vi "3_1_PTLF_Classification_Eval(CPU,GPU).vi"() -> ()   [LabVIEW 2020]
doc: "This example demonstrates the usage of \"Deep Neural Network Accelerator for FPGA\" for Face detection and running for inference on RT targets using FPGA."
uses:
  <vilib>/Ngene/Deep Learning Toolkit/Toolkit/NN_Network/Controls/NN_Device.ctl
  <vilib>/Ngene/Deep Learning Toolkit/Toolkit/NN_Network/Controls/NN_Save_Before_Destroy_Options.ctl
  4973630c-52a8-4b5a-885b-d0de098afee9.vi
  <vilib>/Ngene/Deep Learning Toolkit/Toolkit/NN_Data/subVIs/Get_Data_Vals/2D/NN_Data_Get_ValByRef(2D_SGL).vi
  <vilib>/Ngene/Deep Learning Toolkit/Toolkit/NN_Data/subVIs/Dataset/NN_Variant_to_DVR/2D/NN_Data_Variant_to_DVR(2D_SGL).vi
  <vilib>/Ngene/Deep Learning Toolkit/Toolkit/NN_Data/subVIs/Get_Data_Vals/2D/NN_Data_Get_ValByRef(2D_SGL_idx).vi
  <vilib>/Ngene/Deep Learning Toolkit/Toolkit/NN_Network/API/NN_Set_Input/1D/NN_Set_Input(1D_SGL_idx).vi
  <vilib>/Ngene/Deep Learning Toolkit/Toolkit/NN_Train/Eval_Loss/NN_Eval_Test_Error_Loss/NN_Eval(In1D_Out1D).vi
  <vilib>/Ngene/Deep Learning Toolkit/Toolkit/NN_Train/Eval_Loss/NN_Calc_Cofusion_Matrix/NN_Calc_Confusion_Matrix(In1D_Out1D).vi
  <vilib>/Ngene/Deep Learning Toolkit/Toolkit/Deep_Learning_Toolkit_by_Ngene.lvlib
  <vilib>/ptbypt/NI_PtbyPt.lvlib
panel:
  in  "NN_Device":T1
  in  "Weight File Path":path=path "D:/Ngene/GitHub/deepltk_fpga_examples/3_PTLF_Classification(PXI,sbRIO)/Models/0_PTLF_Classification_Original/PTLF_Classifier_weights_24_11_21__13_37_15.bin"
  in  "Configuration File Path":path=path "D:/Ngene/GitHub/deepltk_fpga_examples/3_PTLF_Classification(PXI,sbRIO)/Models/0_PTLF_Classification_Original/PTLF_Classifier_net_cfg_24_11_21__13_37_15.cfg"
  out "Dataset Size":i32=1200
  out "Loop time(s)":dbl=0.0010359500000049592 format="%#_4p"
  out "Inference time(s)":dbl=0.001025560000061887 format="%#_4p"
  in  "Stop":bool
  out "Iterations":i32=1199
  in  "Dataset":path=path "D:/Ngene/GitHub/deepltk_fpga_examples/3_PTLF_Classification(PXI,sbRIO)/Dataset/Test"
  out "GT":string="Swell"
  out "Pred":string="Sag"
  in  "index":i32=5
  out "Incorectly Classified Sample":sgl[](graph)=[0.419, 0.429, 0.438, 0.446, 0.454, 0.462, 0.469, 0.475, 0.481, 0.487, 0.491, 0.495, 0.499, 0.502, 0.504, 0.506, 0.507, 0.508, 0.508, 0.508, 0.506, 0.505, 0.502, 0.499, 0.496, 0.492, 0.487, 0.482, 0.476, 0.47, 0.463, 0.456, 0.448, 0.439, 0.43, 0.421, 0.411, 0.4, 0.389, 0.378, 0.366, 0.354, 0.341, 0.328, 0.315, 0.301, 0.287, 0.272, 0.257, 0.242, 0.227, 0.211, 0.195, 0.179, 0.163, 0.146, 0.13, 0.113, 0.096, 0.079, 0.061, 0.044, 0.027, 0.01, -0.008, -0.025, -0.043, -0.06, -0.077, -0.094, -0.111, -0.128, -0.145, -0.161, -0.178, -0.194, -0.21, -0.225, -0.241, -0.256, -0.271, -0.285, -0.3, -0.313, -0.327, -0.34, -0.353, -0.365, -0.377, -0.388, -0.399, -0.41, -0.42, -0.429, -0.438, -0.447, -0.455, -0.462, -0.469, -0.652, -0.66, -0.667, -0.673, -0.679, -0.684, -0.688, -0.691, -0.694, -0.695, -0.696, -0.696, -0.695, -0.694, -0.691, -0.688, -0.684, -0.679, -0.674, -0.667, -0.66, -0.652, -0.643, -0.634, -0.624, -0.613, -0.601, -0.589, -0.576, -0.562, -0.548, -0.533, -0.517, -0.501, -0.484, -0.466, -0.449, -0.43, -0.411, -0.392, -0.372, -0.351, -0.331, -0.31, -0.288, -0.266, -0.244, -0.222, -0.199, -0.176, -0.153, -0.13, -0.106, -0.083, -0.059, -0.035, -0.012, 0.012, 0.036, 0.06, 0.083, 0.107, 0.13, 0.154, 0.177, 0.2, 0.222, 0.245, 0.267, 0.289, 0.31, 0.331, 0.352, 0.372, 0.392, 0.412, 0.43, 0.449, 0.467, 0.484, 0.501, 0.517, 0.533, 0.548, 0.562, 0.576, 0.589, 0.601, 0.613, 0.624, 0.634, 0.643, 0.652, 0.66, 0.667, 0.674, 0.679, 0.684, 0.688, 0.691, 0.694, 0.695, 0.696, 0.696, 0.695, 0.694, 0.691, 0.688, 0.684, 0.679, 0.673, 0.667, 0.659, 0.651, 0.643, 0.633, 0.623, 0.612, 0.6, 0.588, 0.575, 0.561, 0.547, 0.532, 0.516, 0.5, 0.483, 0.465, 0.447, 0.429, 0.41, 0.391, 0.371, 0.35, 0.329, 0.308, 0.287, 0.265, 0.243, 0.22, 0.198, 0.175, 0.152, 0.128, 0.105, 0.081, 0.058, 0.034, 0.01, -0.014, -0.037, -0.061, -0.085, -0.108, -0.132, -0.155, -0.178, -0.201, -0.224, -0.246, -0.268, -0.29, -0.311, -0.332, -0.353, -0.373, -0.393, -0.413, -0.432, -0.45, -0.468, -0.485, -0.502, -0.518, -0.534, -0.549, -0.563, -0.577, -0.59, -0.602, -0.614, -0.624, -0.635, -0.644, -0.653, -0.661, -0.668, -0.674, -0.68, -0.684, -0.688, -0.691, -0.694, -0.695, -0.696, -0.696, -0.695, -0.693, -0.691, -0.688, -0.683, -0.679, -0.673, -0.666, -0.659, -0.651, -0.642, -0.633, -0.622, -0.611, -0.6, -0.587, -0.574, -0.56, -0.546, -0.531, -0.515, -0.499, -0.482, -0.464, -0.446, -0.428, -0.409, -0.389, -0.369, -0.349, -0.328, -0.307, -0.286, -0.264, -0.242, -0.219, -0.196, -0.173, -0.15, -0.127, -0.104, -0.08, -0.056, -0.033, -0.009, 0.015, 0.039, 0.063, 0.086, 0.11, 0.133, 0.156, 0.131, 0.148, 0.164, 0.181, 0.197, 0.213, 0.228, 0.244, 0.259, 0.274, 0.288, 0.302, 0.316, 0.329, 0.342, 0.355, 0.367, 0.379, 0.39, 0.401, 0.412, 0.422, 0.431, 0.44, 0.448, 0.456, 0.464, 0.471, 0.477, 0.483, 0.488, 0.492, 0.496, 0.5, 0.503, 0.505, 0.507, 0.508, 0.508, 0.508, 0.507, 0.506, 0.504, 0.502, 0.499, 0.495, 0.491, 0.486, 0.481, 0.475, 0.468, 0.461, 0.454, 0.446, 0.437, 0.428, 0.418, 0.408, 0.398, 0.387, 0.375, 0.363, 0.351, 0.338, 0.325, 0.311, 0.298, 0.283, 0.269, 0.254, 0.239, 0.223, 0.207, 0.192, 0.175, 0.159, 0.142, 0.126, 0.109, 0.092, 0.075, 0.057, 0.04, 0.023, 0.005, -0.012, -0.029, -0.047, -0.064, -0.081, -0.098, -0.115, -0.132, -0.149, -0.165, -0.182, -0.198, -0.214, -0.229, -0.245, -0.26, -0.274, -0.289, -0.303, -0.317, -0.33, -0.343, -0.356, -0.368, -0.38, -0.391, -0.402, -0.412, -0.422, -0.432, -0.44, -0.449, -0.457, -0.464, -0.471, -0.477, -0.483, -0.488, -0.493, -0.497, -0.5, -0.503, -0.505, -0.507, -0.508, -0.508, -0.508, -0.507, -0.506, -0.504, -0.502, -0.499, -0.495, -0.491, -0.486, -0.48, -0.474, -0.468, -0.461, -0.453, -0.445, -0.437, -0.427, -0.418, -0.408, -0.397, -0.386, -0.375, -0.363, -0.35, -0.337, -0.324, -0.311, -0.297, -0.282, -0.268, -0.253, -0.238, -0.222, -0.207, -0.191, -0.174, -0.158, -0.141, -0.125, -0.108, -0.091, -0.074, -0.056, -0.039, -0.022, -0.004, 0.013, 0.03, 0.048, 0.065, 0.082, 0.099, 0.116, 0.133, 0.15, 0.166, 0.183, 0.199, 0.214, 0.23, 0.245, 0.261, 0.275, 0.29, 0.304, 0.318, 0.331, 0.344, 0.356, 0.369, 0.38, 0.392, 0.402, 0.413, 0.423, 0.432, 0.441, 0.449, 0.457, 0.465, 0.471, 0.478, 0.483, 0.488, 0.493, 0.497, 0.5, 0.503, 0.505, 0.507, 0.508, 0.508, 0.508, 0.507, 0.506, 0.504, 0.501, 0.498, 0.495, 0.49, 0.485, 0.48, 0.474, 0.468, 0.46, 0.453, 0.445, 0.436, 0.427, 0.417, 0.407, 0.396, 0.385, 0.374, 0.362, 0.349, 0.337, 0.323, 0.31, 0.296, 0.282, 0.267, 0.252, 0.237, 0.221, 0.206, 0.19, 0.173, 0.157, 0.14, 0.124, 0.107, 0.09, 0.072, 0.055, 0.038, 0.021, 0.003, -0.014, -0.031, -0.049, -0.066, -0.083, -0.1, -0.117, -0.134, -0.151, -0.167, -0.183, -0.2, -0.215, -0.231, -0.246, -0.261, -0.276, -0.291, -0.305, -0.318, -0.332, -0.345, -0.357, -0.369, -0.381, -0.392, -0.403, -0.413, -0.423, -0.433, -0.442, -0.45, -0.458, -0.465, -0.472, -0.478, -0.484, -0.489, -0.493, -0.497, -0.5, -0.503, -0.505, -0.507, -0.508, -0.508, -0.508, -0.507, -0.506, -0.504, -0.501, -0.498, -0.494, -0.49, -0.485, -0.48, -0.474, -0.467, -0.46, -0.452, -0.444, -0.436, -0.426, -0.417, -0.406, -0.396, -0.385, -0.373, -0.361, -0.349, -0.336, -0.323, -0.309, -0.295, -0.281, -0.266, -0.251, -0.236, -0.22, -0.205, -0.189, -0.172, -0.156, -0.139, -0.123, -0.106, -0.089, -0.071, -0.054, -0.037, -0.02, -0.002, 0.015, 0.032, 0.05, 0.067, 0.084, 0.101, 0.118, 0.135, 0.152, 0.168, 0.184, 0.201, 0.216, 0.232, 0.247, 0.262, 0.277, 0.291, 0.305, 0.319, 0.332, 0.345, 0.358, 0.37, 0.382, 0.393, 0.404, 0.414, 0.424, 0.433, 0.442, 0.45, 0.458, 0.465, 0.472, 0.478, 0.484, 0.489, 0.493, 0.497, 0.5, 0.503, 0.505, 0.507, 0.508, 0.508, 0.508, 0.507, 0.506, 0.504, 0.501, 0.498, 0.494, 0.49, 0.485, 0.479, 0.473, 0.467, 0.46, 0.452, 0.444, 0.435, 0.426, 0.416, 0.406, 0.395, 0.384, 0.372, 0.36, 0.348, 0.335, 0.322, 0.308, 0.294, 0.28, 0.265, 0.25, 0.235, 0.219, 0.204, 0.188, 0.171, 0.155, 0.138, 0.122, 0.105, 0.088, 0.07, 0.053, 0.036, 0.019, 0.001, -0.016, -0.034, -0.051, -0.068, -0.085, -0.102, -0.119, -0.136, -0.153, -0.169, -0.185, -0.201, -0.217, -0.233, -0.248, -0.263, -0.278, -0.292, -0.306, -0.32, -0.333, -0.346, -0.359, -0.371, -0.382, -0.394, -0.404, -0.415, -0.424, -0.434, -0.443, -0.451, -0.459, -0.466, -0.472, -0.479, -0.484, -0.489, -0.494, -0.497, -0.501, -0.503, -0.505, -0.507, -0.508, -0.508, -0.508, -0.507, -0.506, -0.504, -0.501, -0.498, -0.494, -0.49, -0.485, -0.479, -0.473, -0.466, -0.459, -0.451, -0.443, -0.434, -0.425, -0.415, -0.405, -0.394, -0.383, -0.372, -0.36, -0.347, -0.334, -0.321, -0.307, -0.293, -0.279, -0.264, -0.249, -0.234, -0.219, -0.203, -0.187, -0.17, -0.154, -0.137, -0.121, -0.104, -0.087, -0.069, -0.052, -0.035, -0.018, -0.0, 0.017, 0.035, 0.052, 0.069, 0.086, 0.103, 0.12, 0.137, 0.154, 0.17, 0.186, 0.202, 0.218, 0.234, 0.249, 0.264, 0.279, 0.293, 0.307, 0.321, 0.334, 0.347, 0.359, 0.371, 0.383, 0.394, 0.405, 0.415, 0.425, 0.434, 0.443, 0.451, 0.459, 0.466, 0.473, 0.479, 0.484, 0.489, 0.494, 0.498, 0.501, 0.504, 0.506, 0.507, 0.508, 0.508, 0.508, 0.507, 0.505, 0.503, 0.501, 0.497, 0.494, 0.489, 0.484, 0.479, 0.473, 0.466, 0.459, 0.451, 0.443, 0.434, 0.425, 0.415, 0.405, 0.394, 0.383, 0.371, 0.359, 0.346, 0.333, 0.32, 0.307, 0.292, 0.278, 0.263, 0.248, 0.233, 0.218, 0.202, 0.186, 0.169, 0.153, 0.136, 0.12, 0.103, 0.086, 0.068, 0.051, 0.034, 0.016, -0.001, -0.018, -0.036, -0.053, -0.07, -0.087, -0.104, -0.121, -0.138, -0.155, -0.171, -0.187, -0.203, -0.219, -0.235, -0.25, -0.265, -0.28, -0.294, -0.308, -0.322, -0.335, -0.348, -0.36, -0.372, -0.384, -0.395, -0.406, -0.416, -0.426, -0.435, -0.444, -0.452, -0.459, -0.467, -0.473, -0.479, -0.485, -0.49, -0.494, -0.498, -0.501, -0.504, -0.506, -0.507, -0.508, -0.508, -0.508, -0.507, -0.505, -0.503, -0.501, -0.497, -0.493, -0.489, -0.484, -0.478, -0.472, -0.465, -0.458, -0.45, -0.442, -0.433, -0.424, -0.414, -0.404, -0.393, -0.382, -0.37, -0.358, -0.346, -0.333, -0.319, -0.306, -0.292, -0.277, -0.263, -0.248, -0.232, -0.217, -0.201, -0.185, -0.168, -0.152, -0.135, -0.119, -0.102, -0.084, -0.067, -0.05, -0.033, -0.015, 0.002, 0.019, 0.037, 0.054, 0.071, 0.088, 0.105, 0.122, 0.139, 0.156, 0.172, 0.188, 0.204, 0.22, 0.236, 0.251, 0.266, 0.28, 0.295, 0.309, 0.322, 0.336, 0.348, 0.361, 0.373, 0.384, 0.396, 0.406, 0.416, 0.426, 0.435, 0.444, 0.452, 0.46, 0.467, 0.474, 0.48, 0.485, 0.49, 0.494, 0.498, 0.501, 0.504, 0.506, 0.507, 0.508, 0.508, 0.508, 0.507, 0.505, 0.503, 0.5, 0.497, 0.493, 0.489, 0.484, 0.478, 0.472, 0.465, 0.458, 0.45, 0.442, 0.433, 0.423, 0.414, 0.403, 0.393, 0.381, 0.37, 0.357, 0.345, 0.332, 0.319, 0.305, 0.291, 0.276, 0.262, 0.247, 0.231, 0.216, 0.2, 0.184, 0.167, 0.151, 0.134, 0.117, 0.101, 0.083, 0.066, 0.049, 0.032, 0.014, -0.003, -0.02, -0.038, -0.055, -0.072, -0.089, -0.106, -0.123, -0.14, -0.157, -0.173, -0.189, -0.205, -0.221, -0.237, -0.252, -0.267, -0.281, -0.296, -0.31, -0.323, -0.336, -0.349, -0.362, -0.374, -0.385, -0.396, -0.407, -0.417, -0.427, -0.436, -0.445, -0.453, -0.46, -0.467, -0.474, -0.48, -0.485, -0.49, -0.495, -0.498, -0.501, -0.504, -0.506, -0.507, -0.508, -0.508, -0.508, -0.507, -0.505, -0.503, -0.5, -0.497, -0.493, -0.488, -0.483, -0.478, -0.471, -0.465, -0.457, -0.45, -0.441, -0.432, -0.423, -0.413, -0.403, -0.392, -0.381, -0.369, -0.357, -0.344, -0.331, -0.318, -0.304, -0.29, -0.276, -0.261, -0.246, -0.23, -0.215, -0.199, -0.183, -0.166, -0.15, -0.133, -0.116, -0.1, -0.082, -0.065, -0.048, -0.031, -0.013, 0.004, 0.021, 0.039, 0.056, 0.073, 0.09, 0.107, 0.124, 0.141, 0.158, 0.174, 0.19, 0.206, 0.222, 0.238, 0.253, 0.268, 0.282, 0.297, 0.31, 0.324, 0.337, 0.35, 0.362, 0.374, 0.386, 0.397, 0.408, 0.418, 0.427, 0.436, 0.445, 0.453, 0.461, 0.468, 0.474, 0.48, 0.486, 0.491, 0.495, 0.498, 0.502, 0.504, 0.506, 0.507, 0.508, 0.508, 0.508, 0.507, 0.505, 0.503, 0.5, 0.497, 0.493, 0.488, 0.483, 0.477, 0.471, 0.464, 0.457, 0.449, 0.441, 0.432, 0.422, 0.412, 0.402, 0.391, 0.38, 0.368, 0.356, 0.343, 0.33, 0.317, 0.303, 0.289, 0.275, 0.26, 0.245, 0.229, 0.214, 0.198, 0.182, 0.166, 0.149, 0.132, 0.115, 0.098, 0.081, 0.064, 0.047, 0.03, 0.012, -0.005, -0.022, -0.04, -0.057, -0.074, -0.091, -0.108, -0.125, -0.142, -0.159, -0.175, -0.191, -0.207, -0.223, -0.238, -0.254, -0.269, -0.283, -0.297, -0.311, -0.325, -0.338, -0.351, -0.363, -0.375, -0.387, -0.398, -0.408, -0.418, -0.428, -0.437, -0.446, -0.454, -0.461, -0.468, -0.475, -0.481, -0.486, -0.491, -0.495, -0.499, -0.502, -0.504, -0.506, -0.507, -0.508, -0.508, -0.508, -0.507, -0.505, -0.503, -0.5, -0.496, -0.492, -0.488, -0.483, -0.477, -0.471, -0.464, -0.456, -0.449, -0.44, -0.431, -0.422, -0.412, -0.401, -0.391, -0.379, -0.367, -0.355, -0.343, -0.33, -0.316, -0.302, -0.288, -0.274, -0.259, -0.244, -0.228, -0.213, -0.197, -0.181, -0.165, -0.148, -0.131, -0.114, -0.097, -0.08, -0.063, -0.046, -0.029, -0.011, 0.006, 0.023, 0.041, 0.058, 0.075, 0.092, 0.109, 0.126, 0.143, 0.16, 0.176, 0.192, 0.208, 0.224, 0.239, 0.255, 0.269, 0.284, 0.298, 0.312, 0.326, 0.339, 0.351, 0.364, 0.376, 0.387, 0.398, 0.409, 0.419, 0.428, 0.438, 0.446, 0.454, 0.462, 0.469, 0.475, 0.481, 0.486, 0.491, 0.495, 0.499, 0.502, 0.504, 0.506, 0.507, 0.508, 0.508, 0.508, 0.507, 0.505, 0.503, 0.5, 0.496, 0.492, 0.487, 0.482, 0.477, 0.47, 0.463, 0.456, 0.448, 0.44, 0.431, 0.421, 0.411, 0.401, 0.39, 0.378, 0.367, 0.354, 0.342, 0.329, 0.315, 0.302, 0.287, 0.273, 0.258, 0.243, 0.228, 0.212, 0.196, 0.18, 0.164, 0.147, 0.13, 0.113, 0.096, 0.079, 0.062, 0.045, 0.028, 0.01, -0.007, -0.025, -0.042, -0.059, -0.076, -0.093, -0.11, -0.127, -0.144, -0.161, -0.177, -0.193, -0.209, -0.225, -0.24, -0.255, -0.27, -0.285, -0.299, -0.313, -0.326, -0.34, -0.352, -0.365, -0.376, -0.388, -0.399, -0.409, -0.419, -0.429, -0.438, -0.447, -0.455, -0.462, -0.469, -0.475, -0.481, -0.487, -0.491, -0.495, -0.499, -0.502, -0.504, -0.506, -0.507, -0.508, -0.508, -0.508, -0.506, -0.505, -0.502, -0.499, -0.496, -0.492, -0.487, -0.482, -0.476, -0.47, -0.463, -0.456, -0.448, -0.439, -0.43, -0.421, -0.411, -0.4, -0.389, -0.378, -0.366, -0.354, -0.341, -0.328, -0.314, -0.301, -0.286, -0.272, -0.257, -0.242, -0.227, -0.211, -0.195, -0.179, -0.163, -0.146, -0.129, -0.112, -0.095, -0.078, -0.061, -0.044, -0.027, -0.009, 0.008, 0.026, 0.043, 0.06, 0.077, 0.094, 0.111, 0.128, 0.145, 0.162, 0.178, 0.194, 0.21, 0.226, 0.241, 0.256, 0.271, 0.286, 0.3, 0.314, 0.327, 0.34, 0.353, 0.365, 0.377, 0.389, 0.4, 0.41, 0.42, 0.43, 0.439, 0.447, 0.455, 0.463, 0.469, 0.476, 0.482, 0.487, 0.492, 0.496, 0.499, 0.502, 0.505, 0.506, 0.508, 0.508, 0.508, 0.508, 0.506, 0.505, 0.502, 0.499, 0.496, 0.492, 0.487, 0.482, 0.476, 0.469, 0.463, 0.455, 0.447, 0.439, 0.43, 0.42, 0.41, 0.399, 0.389, 0.377, 0.365, 0.353, 0.34, 0.327, 0.314, 0.3, 0.286, 0.271, 0.256, 0.241, 0.226, 0.21, 0.194, 0.178, 0.162, 0.145, 0.128, 0.111, 0.094, 0.077, 0.06, 0.043, 0.025, 0.008, -0.009, -0.027, -0.044, -0.061, -0.078, -0.095, -0.112, -0.129, -0.146, -0.163, -0.179, -0.195, -0.211, -0.227, -0.242, -0.257, -0.272, -0.287, -0.301, -0.315, -0.328, -0.341, -0.354, -0.366, -0.378, -0.389, -0.4, -0.411, -0.421, -0.43, -0.439, -0.448, -0.456, -0.463, -0.47, -0.476, -0.482, -0.487, -0.492, -0.496, -0.499, -0.502, -0.505, -0.506, -0.508, -0.508, -0.508, -0.507, -0.506, -0.504, -0.502, -0.499, -0.495, -0.491, -0.487, -0.481, -0.475, -0.469, -0.462, -0.455, -0.447, -0.438, -0.429, -0.419, -0.409, -0.399, -0.388, -0.376, -0.364, -0.352, -0.339, -0.326, -0.313, -0.299, -0.285, -0.27, -0.255, -0.24, -0.225, -0.209, -0.193, -0.177, -0.161, -0.144, -0.127, -0.11, -0.093, -0.076, -0.059, -0.042, -0.024, -0.007, 0.01, 0.028, 0.045, 0.062, 0.079, 0.097, 0.114, 0.13, 0.147, 0.164, 0.18, 0.196, 0.212, 0.228, 0.243, 0.258, 0.273, 0.287, 0.302, 0.315, 0.329, 0.342, 0.354, 0.367, 0.379, 0.39, 0.401, 0.411, 0.421, 0.431, 0.44, 0.448, 0.456, 0.463, 0.47, 0.477, 0.482, 0.488, 0.492, 0.496, 0.5, 0.503, 0.505, 0.507, 0.508, 0.508, 0.508, 0.507, 0.506, 0.504, 0.502, 0.499, 0.495, 0.491, 0.486, 0.481, 0.475, 0.469, 0.462, 0.454, 0.446, 0.437, 0.428, 0.419, 0.409, 0.398, 0.387, 0.376, 0.364, 0.351, 0.339, 0.326, 0.312, 0.298, 0.284, 0.269, 0.254, 0.239, 0.224, 0.208, 0.192, 0.176, 0.16, 0.143, 0.126, 0.109, 0.092, 0.075, 0.058, 0.041, 0.023, 0.006, -0.011, -0.029, -0.046, -0.063, -0.08, -0.098, -0.115, -0.131, -0.148, -0.165, -0.181, -0.197, -0.213, -0.229, -0.244, -0.259, -0.274, -0.288, -0.302, -0.316, -0.33, -0.343, -0.355, -0.367, -0.379, -0.391, -0.401, -0.412, -0.422, -0.431, -0.44, -0.449, -0.456, -0.464, -0.471, -0.477, -0.483, -0.488, -0.492, -0.496, -0.5, -0.503, -0.505, -0.507, -0.508, -0.508, -0.508, -0.507, -0.506, -0.504, -0.502, -0.499, -0.495, -0.491, -0.486, -0.481, -0.475, -0.468, -0.461, -0.454, -0.446, -0.437, -0.428, -0.418, -0.408, -0.398, -0.386, -0.375, -0.363, -0.351, -0.338, -0.325, -0.311, -0.297, -0.283, -0.268, -0.254, -0.238, -0.223, -0.207, -0.191, -0.175, -0.159, -0.142, -0.125, -0.108, -0.091, -0.074, -0.057, -0.04, -0.022, -0.005, 0.012, 0.03, 0.047, 0.064, 0.081]
  out "Confusion Matrix (Table)":string[][](table)=[["200", "0", "0", "0", "0", "0", "1.0000"], ["0", "199", "0", "1", "0", "0", "0.9950"], ["0", "0", "200", "0", "0", "0", "1.0000"], ["0", "0", "1", "197", "2", "0", "0.9850"], ["0", "0", "1", "23", "176", "0", "0.8800"], ["0", "0", "0", "0", "0", "200", "1.0000"], ["1.0000", "1.0000", "0.9901", "0.8914", "0.9888", "1.0000", ""]]
  out "Error":sgl=0.023333333
  out "Loss":sgl=0.061028734
  # "Overview: This VI is designed to evaluate (measure the accuracy of) the model when executed on CPU or GPU.\nRequirements: \n•DeepLTK - Deep Learning Toolkit for LabVIEW (https://www.ngene.co/deep-learning-toolkit-for-labview)\nInstructions:\n1.\tProvide the path to the dataset to be evaluated at Dataset control. \n2.\tProvide the \"Network Configuration File Path\" and \"Weight File Path\" generated by 1_PTLF_Classification_Training.vi or sample from project (locted in \"Models\\1_PTLF_Classification_Original\" folder.\n3.Use NN_Device to specify the device (CPU or GPU) for execution. GPU is applicable only for 64-bit LabVIEW.\n4. Run the VI with the default remaining settings.\n5. Observe mersured accuracy at Loss, Error and Confusion Matrix indicators, and analyze Incorectly Classified Sample by selecting samples with help of index control.\n6. Press the Stop button to stop the VI. \nMore Examples: https://github.com/ngenehub/deepltk_fpga_examples"
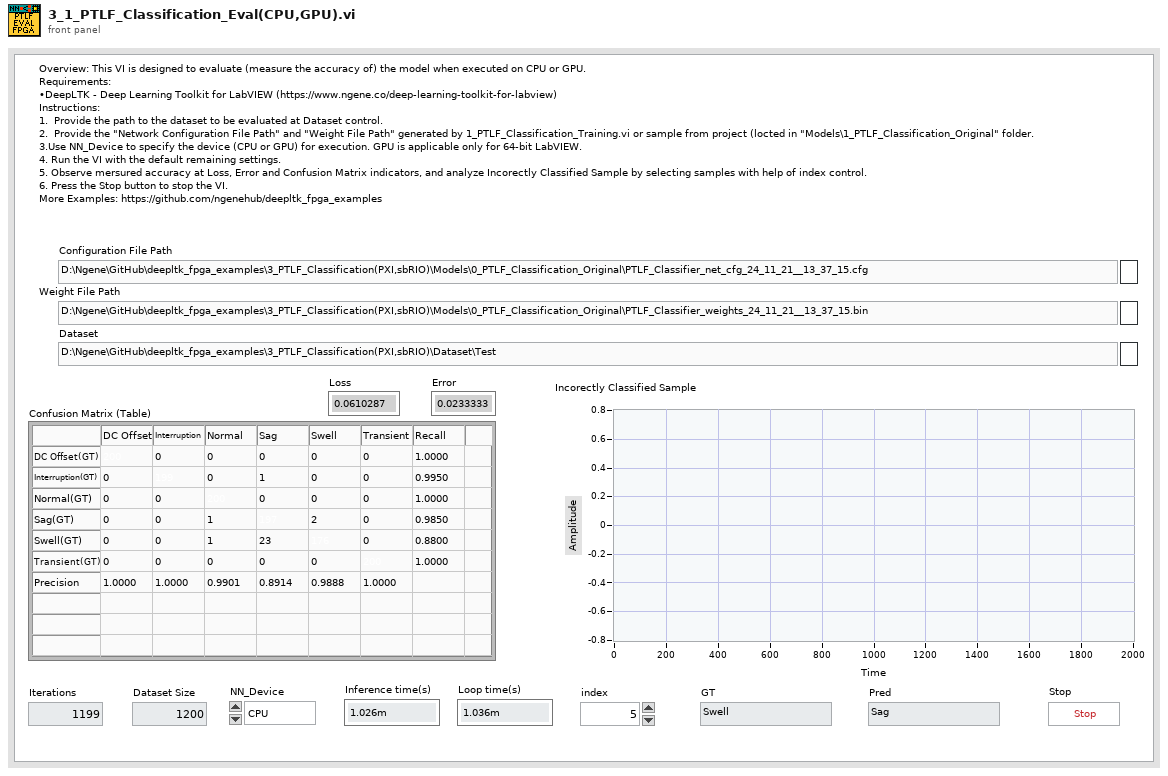
[diagram p1: front panel]
types:
  T1 = typedef "Deep_Learning_Toolkit_by_Ngene.lvlib/NN_Device.ctl" = enum16{"CPU", "GPU"}
  T2 = typedef "Deep_Learning_Toolkit_by_Ngene.lvlib/NN_Save_Before_Destroy_Options.ctl" = cluster{"CFG?":bool, "Weights?":bool, "Render?":bool}
  T3 = typedef "Deep_Learning_Toolkit_by_Ngene.lvlib/NN_DataSets_All(In1D_Out1D).ctl" = cluster{"Train":T4, "Validation":T4, "Test":T4}
  T4 = typedef "Deep_Learning_Toolkit_by_Ngene.lvlib/NN_DataSet(In1D_Out1D).ctl" = cluster{"Inputs Ref.":variant, "Outputs Ref.":T5, "Dims_In":i32, "Dataset_Size":i32, "Dims_Out":i32, "Labels":string[], "File Paths":path[]}
  T5 = typedef "Deep_Learning_Toolkit_by_Ngene.lvlib/NN_Data_ref(2D_SGL).ctl" = refnum<data-value>
  T6 = typedef "Deep_Learning_Toolkit_by_Ngene.lvlib/NN_Config_Params.ctl" = cluster{"Name":string, "mBatch":i32, "NN_Train_Params":T7, "LR_Decay_Policy":T10, "Labels":string[], "Loss":T12}
  T7 = typedef "Deep_Learning_Toolkit_by_Ngene.lvlib/NN_Train_Params.ctl" = cluster{"Optimizer":T8, "Beta_1":sgl, "Beta_2":sgl, "Weight Decay(L1)":sgl, "Weight Decay(L2)":sgl, "Data_Sampling":T9}
  T8 = typedef "Deep_Learning_Toolkit_by_Ngene.lvlib/NN_Train_Optimizer.ctl" = enum16{"SGD", "Adam", "Adagrad", "Adadelta", "RMSProp", "Nesterov"}
  T9 = typedef "Deep_Learning_Toolkit_by_Ngene.lvlib/NN_Train_Data_Sampling.ctl" = enum16{"Random", "Sequential"}
  T10 = typedef "Deep_Learning_Toolkit_by_Ngene.lvlib/NN_LR_Policy_Cfg.ctl" = cluster{"Policy_Type":T11, "LR0":dbl, "k":sgl, "WarmUp_Policy":enum16{"Step", "Ramp"}, "WarmUp_Iter":i32, "WarmUp_Ratio":sgl}
  T11 = typedef "Deep_Learning_Toolkit_by_Ngene.lvlib/NN_LR_Policy_Type.ctl" = enum16{"Manual", "Step", "Exp", "1/t"}
  T12 = typedef "Deep_Learning_Toolkit_by_Ngene.lvlib/NN_Loss_Config_Params.ctl" = cluster{"Loss_Type":T13, "Loss_Conf_Params":variant}
  T13 = typedef "Deep_Learning_Toolkit_by_Ngene.lvlib/NN_Loss_Type.ctl" = enum16{"None", "MSE", "CrossEntropy", "YOLO_v2", "YOLO_v4"}
  T14 = typedef "Deep_Learning_Toolkit_by_Ngene.lvlib/NN_Layer_Config_Params.ctl" = cluster{"Layer_Type":T15, "Layer_Conf_Params":variant, "Input Layers":string[]}
  T15 = typedef "Deep_Learning_Toolkit_by_Ngene.lvlib/NN_Layer_Type.ctl" = enum16{"Input1D", "Input3D", "Conv1D", "Conv2D", "Conv2D_Adv", "MaxPool", "AvgPool", "UpSample", "DropOut3D", "ShortCut", "Concat", "SoftMax3D", "FC", "DropOut", "Softmax", "Flatten", "YOLO_v2", "YOLO_v4", "Activation", "BatchNormalization", "Unsupported"}
  T16 = typedef "Deep_Learning_Toolkit_by_Ngene.lvlib/NN.ctl" = cluster{"Name":string, "No of Layers":i32, "mBatch":i32, "Layers":T17[], "Dimty":T18, "Dims_In":T19, "Dims_Out":T19, "Working_Dir":path, "Train?":bool, "Train_Params":T7, "LR_Update_Policy":T10, "Session Data":T20, "Ground_truth":T21, "NNg_hdls":T22, "NN_Device":T1, "GPU Id":i32, "Labels":string[], "Receptive Field":T23[], "Loss_Type":T13, "Loss_Cfg_Prms":variant, "NNG_WS":T24}
  T17 = typedef "Deep_Learning_Toolkit_by_Ngene.lvlib/NN_Layer_ref.ctl" = refnum<data-value>
  T18 = typedef "Deep_Learning_Toolkit_by_Ngene.lvlib/NN_In_Out_Dim-ty.ctl" = enum8{"In1D_Out1D", "In3D_Out1D", "In3D_Out3D", "In3D_OutBBox"}
  T19 = typedef "Deep_Learning_Toolkit_by_Ngene.lvlib/NN_Dims(C,H,W).ctl" = cluster{"C":i32, "H":i32, "W":i32}
  T20 = typedef "Deep_Learning_Toolkit_by_Ngene.lvlib/NN_Train_Session_Data.ctl" = cluster{"Epochs":sgl, "Tot_Iter":i32, "LR":sgl, "LR_iter":i32}
  T21 = typedef "Deep_Learning_Toolkit_by_Ngene.lvlib/NN_Ground_truth.ctl" = cluster{"Y":variant}
  T22 = typedef "Deep_Learning_Toolkit_by_Ngene.lvlib/nng_cuda_handles.ctl" = cluster{"cudnn":u64, "cublas":u64, "stream":u64, "curand":u64}
  T23 = typedef "Deep_Learning_Toolkit_by_Ngene.lvlib/NN_Dims(V,H).ctl" = cluster{"V":i32, "H":i32}
  T24 = typedef "Deep_Learning_Toolkit_by_Ngene.lvlib/NNG_WS.ctl" = cluster{"NNG_WS_Mem":T25, "Max_WS_Size":i64}
  T25 = typedef "Deep_Learning_Toolkit_by_Ngene.lvlib/NNg_WS_Mem_DVR.ctl" = refnum<data-value>
  T26 = typedef "Deep_Learning_Toolkit_by_Ngene.lvlib/NN_Layer.ctl" = cluster{"Name":string, "Layer_Data":variant, "Layer_Type":T15, "Dims_In":T19, "Layers_In":variant, "Dims_Out":T19, "Layers_Out":variant, "Metrics":T27, "GPU_Data":variant, "mBatch":i32, "NN_Device":T1, "NNg_hdls":T22, "Train?":bool, "Dimty":T28, "RecptField":T29}
  T27 = typedef "Deep_Learning_Toolkit_by_Ngene.lvlib/NN_Layer_Metrics.ctl" = cluster{"Data":dbl, "Params":dbl, "Ops":dbl}
  T28 = typedef "Deep_Learning_Toolkit_by_Ngene.lvlib/NN_Layer_Dimty.ctl" = enum16{"1D", "3D"}
  T29 = typedef "Deep_Learning_Toolkit_by_Ngene.lvlib/NN_Layer_RF_State.ctl" = cluster{"Dims":T23, "J":T23}
  T30 = typedef "Deep_Learning_Toolkit_by_Ngene.lvlib/NN_Eval_Params.ctl" = cluster{"Loss":sgl, "Error":sgl}
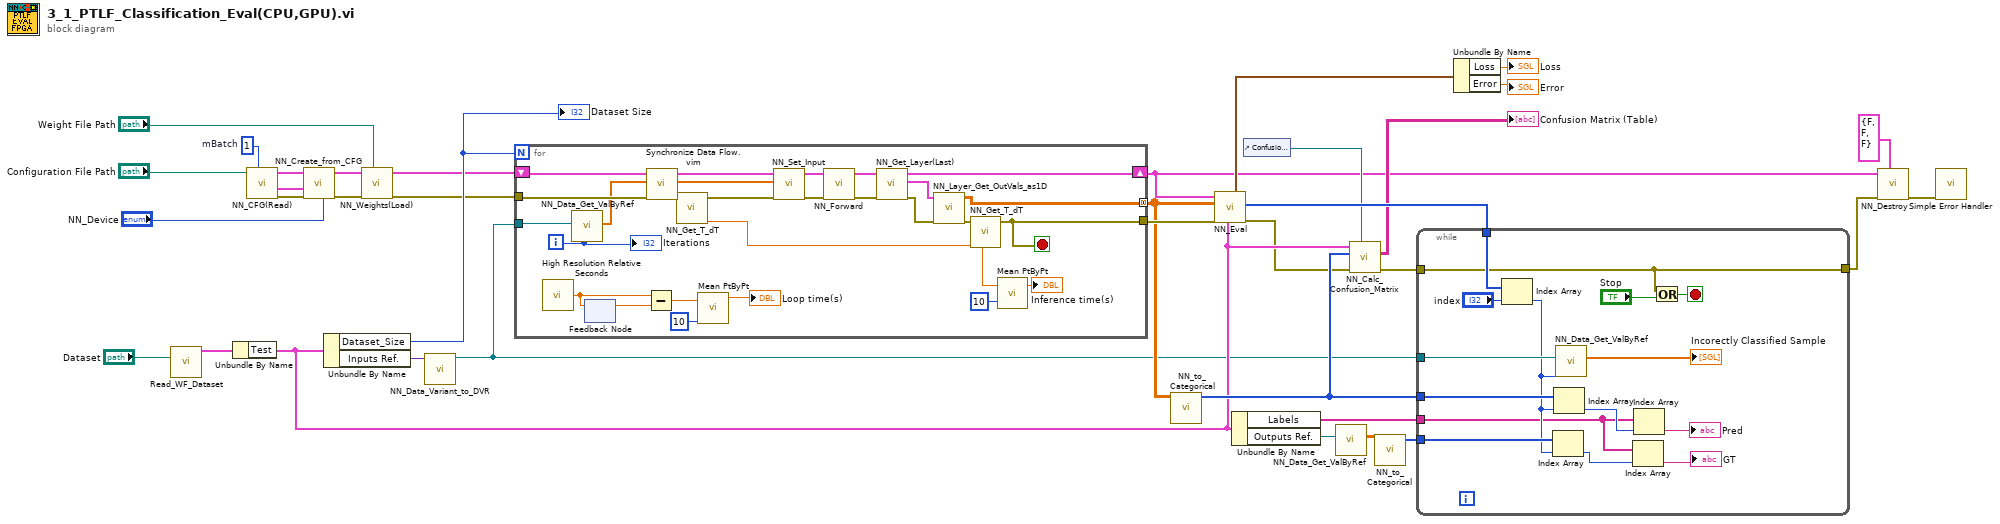
[diagram p0: block diagram]
diagram:
  w7 = 1  # mBatch
  n1 = call "Read_WF_Dataset.vi"("Test dataset path"="Dataset") -> ("NN_Dataset"=w24:T3)  [unwired: 10 in]
  n2 = Unbundle By Name(w24) -> ("Test"=w23:T4)
  n3 = call <vilib>:"NN_CFG(Read).vi"("mBatch"=w7, "CFG file path"="Configuration File Path") -> ("error out"=w10:errorcluster, "Net_Cfg"=w11:T6, "Layer_Cfg"=w9:T14[])  [unwired: 7 in]
  n4 = call <vilib>:"NN_Create_from_CFG.vi"("NN_Device"="NN_Device", "error in (no error)"=w10, "Net_Cfg"=w11, "Layer_Cfg"=w9) -> ("error out"=w12:errorcluster, "NN out"=w8:T16)  [unwired: 6 in]
  n5 = Unbundle By Name(w23) -> ("Dataset_Size"=w16:i32, "Inputs Ref."=w35:variant)
  "Dataset Size" <- w16
  n6 = call <vilib>:"NN_Weights(Load).vi"("Weight File Path"="Weight File Path", "error in (no error)"=w12, "NN in"=w8) -> ("error out"=w3:errorcluster, "NN out"=w4:T16)  [unwired: 7 in]
  n7 = call-poly <vilib>:"NN_Data_Variant_to_DVR.vi"("Inputs Ref."=w35) -> ("DVR(2D_SGL)"=w14:T5)  [unwired: 9 in, 1 out]
  n8 = for {
    N: w16 -> [_]
    shift-right: [w38] -> w15
    shift-left: w4 -> [w54]
    tunnel: w14 -> [w64]
    tunnel: [w59] -> w29 mode=concatenating
    tunnel: [w47] -> w34
    tunnel: w3 -> [w53]
    i -> [w58]
    stop <- w47 stop-if-true
    n9 = call <vilib>:"High Resolution Relative Seconds.vi"() -> ("relative seconds"=w55:dbl)
    n10 = call-poly <vilib>:"NN_Data_Get_ValByRef.vi"("index (row)"=w58, "DVR(2D_SGL)"=w64) -> ("Value(1D_SGL)"=w51:sgl[])  [unwired: 6 in, 1 out]
    n11 = feedback #1() -> (w56:dbl)  [unwired: 1 in]
    n12 = feedback-in #1(w55) -> ()
    n13 = Subtract(x=w55, y=w56) -> (x-y=w57:dbl)
    n14 = call "Synchronize Data Flow.vim"("input 4"=w53, "input 2"=w51, "input 1"=w54) -> ("output 4"=w52:errorcluster, "output 2"=w49:sgl[], "output 1"=w50:T16)  [unwired: 1 in, 1 out]
    n15 = call <vilib>:"NN_Get_T_dT.vi"("error in (no error)"=w52) -> ("T_out"=w46:dbl, "error out"=w48:errorcluster)  [unwired: 6 in, 1 out]
    n16 = call <vilib>:"Mean PtByPt.vi"("x"=w57, "sample length"=10) -> ("mean"=→"Loop time(s)":dbl)  [unwired: 2 in, 1 out]
    n17 = call-poly <vilib>:"NN_Set_Input.vi"("error in (no error)"=w48, "Data_In(1D_SGL)"=w49, "NN In"=w50) -> ("error out"=w62:errorcluster, "NN Out"=w63:T16)  [unwired: 7 in]
    n18 = call <vilib>:"NN_Forward.vi"("error in (no error)"=w62, "NN in"=w63) -> ("error out"=w61:errorcluster, "NN out"=w39:T16)  [unwired: 6 in, 2 out]
    n19 = call <vilib>:"NN_Get_Layer(Last).vi"("error in (no error)"=w61, "NN in"=w39) -> ("error out"=w40:errorcluster, "Last_Layer"=w37:T26, "NN out"=w38:T16)  [unwired: 6 in, 1 out]
    n20 = call <vilib>:"NN_Layer_Get_OutVals_as1D.vi"("error in (no error)"=w40, "Layer"=w37) -> ("error out"=w60:errorcluster, "Out(as1D)"=w59:sgl[][])  [unwired: 8 in]
    n21 = call <vilib>:"NN_Get_T_dT.vi"("T_in"=w46, "error in (no error)"=w60) -> ("error out"=w47:errorcluster, "dT"=w44:dbl)  [unwired: 5 in, 1 out]
    n22 = call <vilib>:"Mean PtByPt.vi"("x"=w44, "sample length"=10) -> ("mean"=→"Inference time(s)":dbl)  [unwired: 2 in, 1 out]
    "Iterations" <- w58
  }
  n23 = call <vilib>:"NN_to_Categorical.vi"("Prediction"=w29) -> ("Label_Idx"=w28:i32[])  [unwired: 10 in]
  n24 = call-poly <vilib>:"NN_Eval.vi"("Dataset"=w23, "error in (no error)"=w34, "Predictions"=w29, "NN in"=w15) -> ("error out"=w19:errorcluster, "Incrct_Class_idx"=w30:i32[], "NN_Eval_Params"=w33:T30)  [unwired: 4 in, 1 out]
  n25 = Unbundle By Name(w23) -> ("Labels"=w13:string[], "Outputs Ref."=w22:T5)
  n26 = control-ref of="Confusion Matrix (Table)"() -> (w20:refnum<vi>)
  n27 = call-poly <vilib>:"NN_Data_Get_ValByRef.vi"("DVR(2D_SGL)"=w22) -> ("Value(2D_SGL)"=w27:sgl[][])  [unwired: 7 in, 1 out]
  n28 = call-poly <vilib>:"NN_Calc_Confusion_Matrix.vi"("Confusion Matrix (Table) ref."=w20, "error in (no error)"=w19, "Predictions"=w28, "Dataset"=w23) -> ("error out"=w18:errorcluster, "Confusion Matrix (Table)"=→"Confusion Matrix (Table)":string[][])  [unwired: 3 in, 3 out]
  n29 = call <vilib>:"NN_to_Categorical.vi"("Prediction"=w27) -> ("Label_Idx"=w26:i32[])  [unwired: 10 in]
  n30 = while {
    tunnel: w14 -> [w79]
    tunnel: w30 -> [w78]
    tunnel: w28 -> [w76]
    tunnel: w26 -> [w75]
    tunnel: [w67] -> w25
    tunnel: w18 -> [w67]
    tunnel: w13 -> [w65]
    stop <- w68 stop-if-true
    n31 = Index Array(array=w78, index="index") -> (element=w74:i32)
    n32 = Index Array(array=w75, index=w74) -> (element=w71:i32)
    n33 = Index Array(array=w76, index=w74) -> (element=w72:i32)
    n34 = call-poly <vilib>:"NN_Data_Get_ValByRef.vi"("index (row)"=w74, "DVR(2D_SGL)"=w79) -> ("Value(1D_SGL)"=→"Incorectly Classified Sample":sgl[])  [unwired: 6 in, 1 out]
    n35 = Index Array(array=w65, index=w71) -> (element=→"GT":string)
    n36 = Index Array(array=w65, index=w72) -> (element=→"Pred":string)
    n37 = Or(x=w67, y="Stop") -> (x .or. y?=w68:bool)
  }
  n38 = Unbundle By Name(w33) -> ("Loss"=→"Loss":sgl, "Error"=→"Error":sgl)
  n39 = call <vilib>:"NN_Destroy.vi"("Save (T, T, T)"=T2 {"CFG?"=FALSE, "Weights?"=FALSE, "Render?"=FALSE}, "error in (no error)"=w25, "NN in"=w15) -> ("error out"=w36:errorcluster)  [unwired: 7 in, 1 out]
  n40 = call <vilib>:"Simple Error Handler.vi"("error in (no error)"=w36) -> ()  [unwired: 4 in, 5 out]
